vi "adapter_extended_audio.vi"(10 "configuration_extended_audio":T1={"chunk"=512, "mixer_mode"=2, "loopback_gain"=1.0, "microphone_gain"=1.0, "profile"=3, "level"=41, "_reserved_0"=0, "_reserved_1"=0}, 11 "path in":path=path "hl2ss_ulm.dll") -> (2 "configuration":u64, 3 "path out":path)   [LabVIEW 2023]
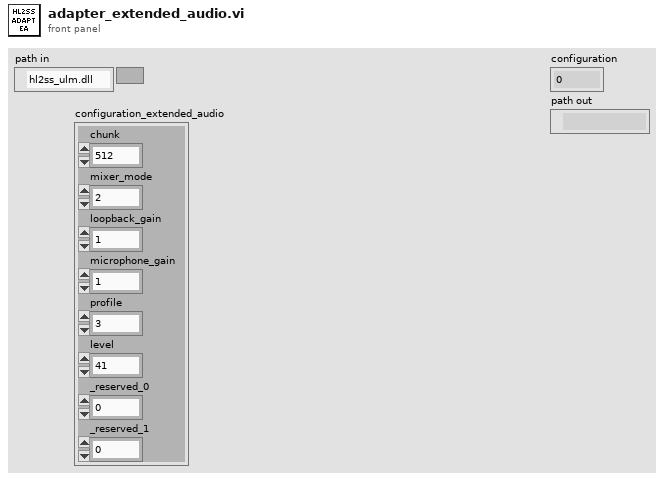
[diagram p1: front panel]
types:
  T1 = cluster{"chunk":u64, "mixer_mode":u32, "loopback_gain":sgl, "microphone_gain":sgl, "profile":u8, "level":u8, "_reserved_0":u8, "_reserved_1":u8}
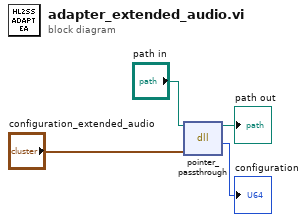
[diagram p0: block diagram]
diagram:
  n1 = dll-call lib="C:/Users/jcds/Documents/GitHub/hl2ss/extensions/client_labview/hl2ss_ulm.dll" fn="pointer_passthrough"(path in="path in", "p"="configuration_extended_audio") -> (path out=→"path out":path, "return type"=→"configuration":u64)  [unwired: 3 in, 1 out]
